vi "CC Script to Table.vi"(8 "error in (no error)":errorcluster, 10 "Line Numbers?":bool, 11 "Script":T1[](array[typedef])) -> (0 "error out":errorcluster, 3 "table":string[][](array[string]))   [LabVIEW 2021]
uses:
  typedefs/CC Script Step.ctl
  typedefs/CC enum Script Action.ctl
  typedefs/CC cluster Object.ctl
  typedefs/CC cluster sidereal rate.ctl
  typedefs/CC cluster RA and DEC.ctl
  typedefs/cc cluster muRA muDEC.ctl
  Telescope/CC cluster Telescope Offsets.ctl
  typedefs/CC cluster Exposure.ctl
  Detector/Detector Class/Detector enum Detector Integration Mode.ctl
  typedefs/CC Dithering.ctl
  typedefs/CC cluster Offset Dithering.ctl
  typedefs/CC Dithering Offsets.ctl
  typedefs/CC cluster Random Dithering.ctl
  typedefs/CC cluster Acquire Parameters.ctl
  typedefs/CC cluster Filter Wheel Parameters.ctl
  Focus/Focus cluster MoveFocus Command Parameters.ctl
  typedefs/CC cluster Pause Parameters.ctl
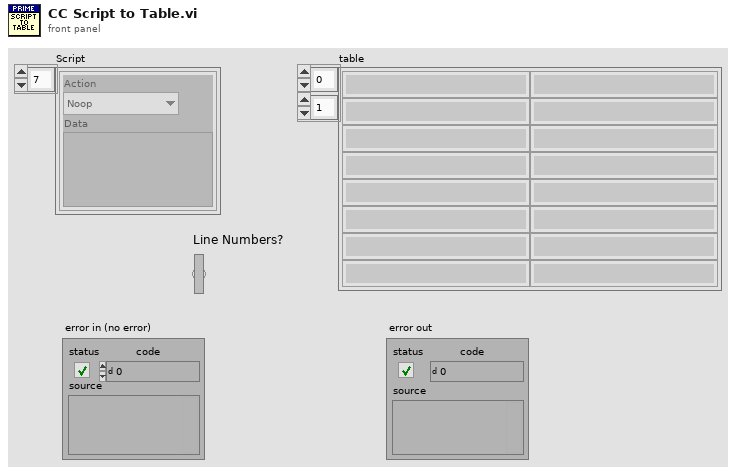
[diagram p1: front panel]
types:
  T1 = typedef "CC Script Step.ctl" = cluster{"Action":T2, "Data":variant}
  T2 = typedef "CC enum Script Action.ctl" = enum16{"Noop", "Define Object", "Define Exposure", "Define Dithering", "Acquire Images", "Set Filter Wheel", "Telescope Home", "Telescope Move", "Telescope RA DEC", "Focus Move Relative", "Focus Move Absolute", "Focus Set Home", "Macro", "Pause", "Ask User", "Define Random Dither"}
  T3 = typedef "CC cluster Object.ctl" = cluster{"Object":cluster{"Name":string}, "Sidereal Rate":T4, "RA and DEC":T5, "muRA muDEC Epoch":T6, "Offsets":T7}
  T4 = typedef "CC cluster sidereal rate.ctl" = cluster{"dRA":dbl, "dDEC":dbl}
  T5 = typedef "CC cluster RA and DEC.ctl" = cluster{"RA":dbl, "DEC":dbl}
  T6 = typedef "cc cluster muRA muDEC.ctl" = cluster{"muRA":dbl, "muDEC":dbl, "Epoch":dbl}
  T7 = typedef "CC cluster Telescope Offsets.ctl" = cluster{"RA":dbl, "DEC":dbl, "ROT":dbl}
  T8 = typedef "CC cluster Exposure.ctl" = cluster{"Mode":T9, "Integration Time":dbl, "Name":string, "Images":i32}
  T9 = typedef "Detector enum Detector Integration Mode.ctl" = enum16{"SSR", "CDS", "MEAN", "MEDIAN", "MODE", "MIIN", "MAX"}
  T10 = typedef "CC Dithering.ctl" = cluster{"Name":string, "Dithering Offsets":T11}
  T11 = typedef "CC cluster Offset Dithering.ctl" = cluster{"Offsets":T12[]}
  T12 = typedef "CC Dithering Offsets.ctl" = cluster{"DEC":dbl, "RA":dbl}
  T13 = typedef "CC cluster Random Dithering.ctl" = cluster{"Count":i32, "Radius":dbl, "Name":string}
  T14 = typedef "CC cluster Acquire Parameters.ctl" = cluster{"Object":string, "Exposure":string, "Dithering":string}
  T15 = typedef "CC cluster Filter Wheel Parameters.ctl" = cluster{"Wheel":i32, "Filter":i32}
  T16 = typedef "Focus cluster MoveFocus Command Parameters.ctl" = cluster{"Motor":i32, "Position":i32}
  T17 = typedef "CC cluster Pause Parameters.ctl" = cluster{"Time (s)":dbl}
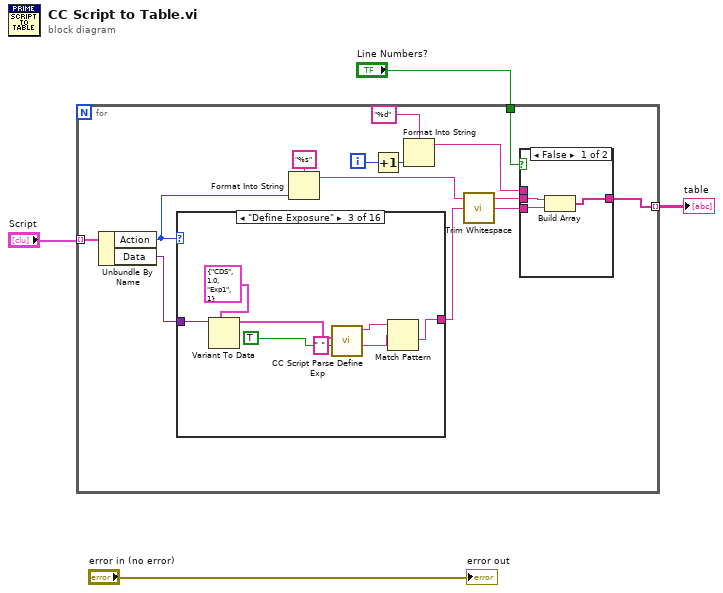
[diagram p0: block diagram]
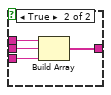
[diagram p2: hidden frame]
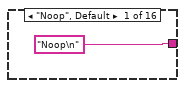
[diagram p3: hidden frame]
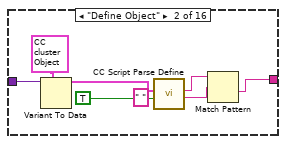
[diagram p4: hidden frame]
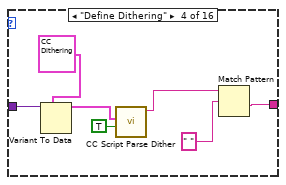
[diagram p5: hidden frame]
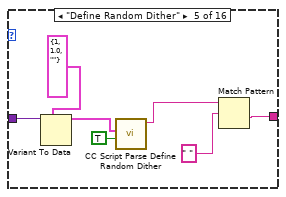
[diagram p6: hidden frame]
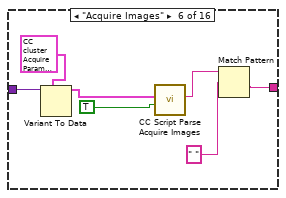
[diagram p7: hidden frame]
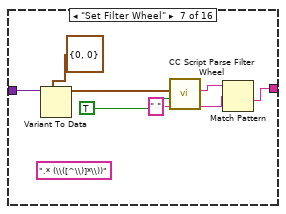
[diagram p8: hidden frame]
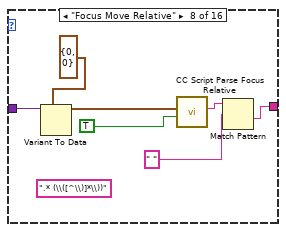
[diagram p9: hidden frame]
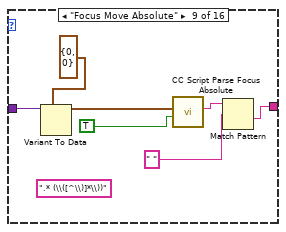
[diagram p10: hidden frame]
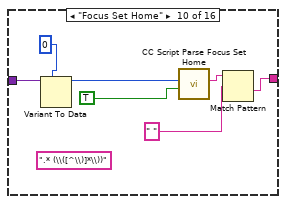
[diagram p11: hidden frame]
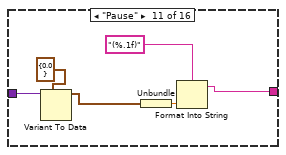
[diagram p12: hidden frame]
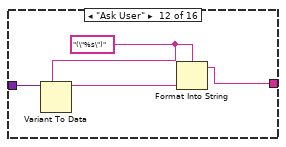
[diagram p13: hidden frame]
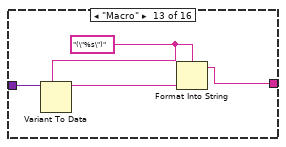
[diagram p14: hidden frame]
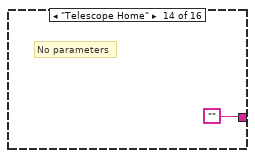
[diagram p15: hidden frame]
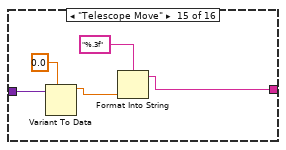
[diagram p16: hidden frame]
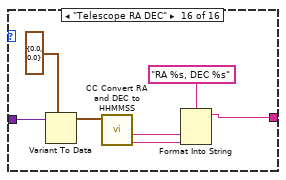
[diagram p17: hidden frame]
diagram:
  n1 = for {
    tunnel: "Script" -> [w17] mode=indexing
    tunnel: [w12] -> w2 mode=indexing
    tunnel: "Line Numbers?" -> [w5]
    i -> [w7]
    n2 = Unbundle By Name(w17) -> ("Action"=w13:T2, "Data"=w14:variant)
    n3 = case shown="\"Define Exposure\"" w13 {
      tunnel: w14 -> [_ w32 w39 w46 w53 w60 w67 w74 w81 w88 w94 w98 w102 _ w108 w115]
      tunnel: ["Noop\n" ("string") w27 w33 w40 w47 w54 w61 w72 w79 w86 w89 w95 w99 "" w104 w113] -> w11
      frame "Noop", Default {
      }
      frame "Define Object" {
        n4 = Variant To Data(type=T3 {"Object"={"Name"=""}, "Sidereal Rate"={"dRA"=0.0, "dDEC"=0.0}, "RA and DEC"={"RA"=0.0, "DEC"=0.0}, "muRA muDEC Epoch"={"muRA"=0.0, "muDEC"=0.0, "Epoch"=0.0}, "Offsets"={"RA"=0.0, "DEC"=0.0, "ROT"=0.0}} ("Object"), Variant=w32) -> (data=w30:T3)  [unwired: 1 in, 1 out]
        n5 = call "CC Script Parse Define.vi"("To String?"=TRUE, "Object in"=w30) -> ("Script"=w28:string)  [unwired: 6 in, 3 out]
        n6 = Match Pattern(string=w28, regular expression=" ") -> (after substring=w27:string)  [unwired: 1 in, 3 out]
      }
      frame "Define Exposure" {
        n7 = Variant To Data(type=T8 {"Mode"=enum."CDS", "Integration Time"=1.0, "Name"="Exp1", "Images"=1} ("Exposure in"), Variant=w39) -> (data=w37:T8)  [unwired: 1 in, 1 out]
        n8 = call "CC Script Parse Define Exp.vi"("To String?"=TRUE, "Exposure in"=w37) -> ("Script String out"=w34:string)  [unwired: 6 in, 3 out]
        n9 = Match Pattern(string=w34, regular expression=" ") -> (after substring=w33:string)  [unwired: 1 in, 3 out]
      }
      frame "Define Dithering" {
        n10 = Variant To Data(type=T10 {"Name"="", "Dithering Offsets"={"Offsets"=[{"DEC"=0.0, "RA"=0.0}, {"DEC"=-10.0, "RA"=-10.0}]}} ("Dithering Offsets in"), Variant=w46) -> (data=w44:T10)  [unwired: 1 in, 1 out]
        n11 = call "CC Script Parse Dither.vi"("To String?"=TRUE, "Dithering in"=w44) -> ("resulting string"=w41:string)  [unwired: 7 in, 2 out]
        n12 = Match Pattern(string=w41, regular expression=" ") -> (after substring=w40:string)  [unwired: 1 in, 3 out]
      }
      frame "Define Random Dither" {
        n13 = Variant To Data(type=T13 {"Count"=1, "Radius"=1.0, "Name"=""} ("Dithering Offsets in"), Variant=w53) -> (data=w51:T13)  [unwired: 1 in, 1 out]
        n14 = call "CC Script Parse Define Random Dither.vi"("To String?"=TRUE, "Random Dither in"=w51) -> ("Script String out"=w48:string)  [unwired: 7 in, 2 out]
        n15 = Match Pattern(string=w48, regular expression=" ") -> (after substring=w47:string)  [unwired: 1 in, 3 out]
      }
      frame "Acquire Images" {
        n16 = Variant To Data(type=T14 {"Object"="Alpha1234", "Exposure"="Exp1", "Dithering"="Dither2"} ("Acquire Parameters in"), Variant=w60) -> (data=w58:T14)  [unwired: 1 in, 1 out]
        n17 = call "CC Script Parse Acquire Images.vi"("To Script?"=TRUE ("To String?"), "Acquire Parameters in"=w58) -> ("Script out"=w55:string)  [unwired: 7 in, 2 out]
        n18 = Match Pattern(string=w55, regular expression=" ") -> (after substring=w54:string)  [unwired: 1 in, 3 out]
      }
      frame "Set Filter Wheel" {
        (unwired) ".* (\\([^\\)]*\\))" ("regular expression")
        n19 = Variant To Data(type=T15 {"Wheel"=0, "Filter"=0} ("Acquire Parameters in"), Variant=w67) -> (data=w65:T15)  [unwired: 1 in, 1 out]
        n20 = call "CC Script Parse Filter Wheel.vi"("To Script?"=TRUE ("To String?"), "Filter Wheel parameters in"=w65) -> ("Script Out"=w62:string)  [unwired: 7 in, 2 out]
        n21 = Match Pattern(string=w62, regular expression=" ") -> (after substring=w61:string)  [unwired: 1 in, 3 out]
      }
      frame "Focus Move Relative" {
        (unwired) ".* (\\([^\\)]*\\))" ("regular expression")
        n22 = Variant To Data(type=T16 {"Motor"=0, "Position"=0} ("Cluster"), Variant=w74) -> (data=w70:T16)  [unwired: 1 in, 1 out]
        n23 = call "CC Script Parse Focus Relative.vi"("To Script?"=TRUE ("To String?"), "Move parm in"=w70) -> ("Script Out"=w68:string)  [unwired: 7 in, 2 out]
        n24 = Match Pattern(string=w68, regular expression=" ") -> (after substring=w72:string)  [unwired: 1 in, 3 out]
      }
      frame "Focus Move Absolute" {
        (unwired) ".* (\\([^\\)]*\\))" ("regular expression")
        n25 = Variant To Data(type=T16 {"Motor"=0, "Position"=0} ("Cluster"), Variant=w81) -> (data=w77:T16)  [unwired: 1 in, 1 out]
        n26 = call "CC Script Parse Focus Absolute.vi"("To Script?"=TRUE ("To String?"), "Move parm in"=w77) -> ("Script Out"=w75:string)  [unwired: 7 in, 2 out]
        n27 = Match Pattern(string=w75, regular expression=" ") -> (after substring=w79:string)  [unwired: 1 in, 3 out]
      }
      frame "Focus Set Home" {
        (unwired) ".* (\\([^\\)]*\\))" ("regular expression")
        n28 = Variant To Data(type=0 ("Motor"), Variant=w88) -> (data=w84:i32)  [unwired: 1 in, 1 out]
        n29 = call "CC Script Parse Focus Set Home.vi"("To Script?"=TRUE ("To String?"), "Set Home parm in"=w84) -> ("Script Out"=w82:string)  [unwired: 7 in, 2 out]
        n30 = Match Pattern(string=w82, regular expression=" ") -> (after substring=w86:string)  [unwired: 1 in, 3 out]
      }
      frame "Pause" {
        n31 = Variant To Data(type=T17 {"Time (s)"=0.0} ("Acquire Parameters in"), Variant=w94) -> (data=w91:T17)  [unwired: 1 in, 1 out]
        n32 = Unbundle(w91) -> ("Time (s)"=w90:dbl)
        n33 = Format Into String(format string="(%.1f)", w90) -> (resulting string=w89:string)  [unwired: 2 in, 1 out]
      }
      frame "Ask User" {
        w97 = "(\"%s\")" ("format string")
        n34 = Variant To Data(type=w97, Variant=w98) -> (data=w96:string)  [unwired: 1 in, 1 out]
        n35 = Format Into String(format string=w97, w96) -> (resulting string=w95:string)  [unwired: 2 in, 1 out]
      }
      frame "Macro" {
        w101 = "(\"%s\")" ("format string")
        n36 = Variant To Data(type=w101, Variant=w102) -> (data=w100:string)  [unwired: 1 in, 1 out]
        n37 = Format Into String(format string=w101, w100) -> (resulting string=w99:string)  [unwired: 2 in, 1 out]
      }
      frame "Telescope Home" {
        # "No parameters"
      }
      frame "Telescope Move" {
        n38 = Variant To Data(type=0.0, Variant=w108) -> (data=w105:dbl)  [unwired: 1 in, 1 out]
        n39 = Format Into String(format string="%.3f", w105) -> (resulting string=w104:string)  [unwired: 2 in, 1 out]
      }
      frame "Telescope RA DEC" {
        n40 = Variant To Data(type=T5 {"RA"=0.0, "DEC"=0.0} ("RA and DEC"), Variant=w115) -> (data=w111:T5)  [unwired: 1 in, 1 out]
        n41 = call "CC Convert RA and DEC to HHMMSS.vi"("RA and DEC"=w111) -> ("DEC String"=w109:string, "RA String"=w110:string)  [unwired: 7 in, 2 out]
        n42 = Format Into String(format string="RA %s, DEC %s", w110, w109) -> (resulting string=w113:string)  [unwired: 2 in, 1 out]
      }
    }
    n43 = Format Into String(format string="%s", w13) -> (resulting string=w15:string)  [unwired: 2 in, 1 out]
    n44 = Increment(x=w7) -> (x+1=w8:i32)
    n45 = Format Into String(format string="%d", w8) -> (resulting string=w6:string)  [unwired: 2 in, 1 out]
    n46 = call <vilib>:"Trim Whitespace.vi"("string"=w11) -> ("trimmed string"=w10:string)  [unwired: 1 in]
    n47 = case shown="False" w5 {
      tunnel: w15 -> [w19 w24]
      tunnel: [w18 w23] -> w12
      tunnel: w10 -> [w20 w22]
      tunnel: w6 -> [_ w21]
      frame False {
        n48 = Build Array(w19, w20) -> (w18:string[])
      }
      frame True {
        n49 = Build Array(w21, w24, w22) -> (w23:string[])
      }
    }
  }
  "table" <- w2
  "error out" <- "error in (no error)"
